vi "Read Modified.vi"(8 "error in (no error)":errorcluster, 11 "LabVIEW-Config In":refnum<class "LabVIEW-Config.lvclass">) -> (0 "error out":errorcluster, 2 "Modified?":bool, 3 "LabVIEW-Config Out":refnum<class "LabVIEW-Config.lvclass">)   [LabVIEW 2017, in "LabVIEW-Config.lvlib" / "LabVIEW-Config.lvclass"]
uses:
  LabVIEW-Config.lvclass
  LabVIEW-Config.lvclass/LabVIEW-Config.ctl
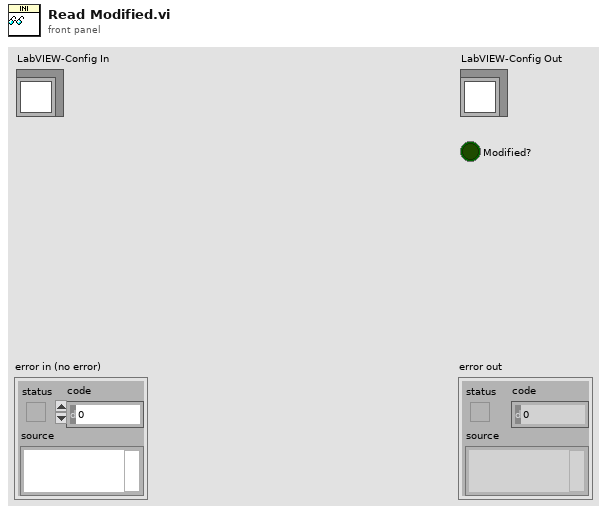
[diagram p1: front panel]
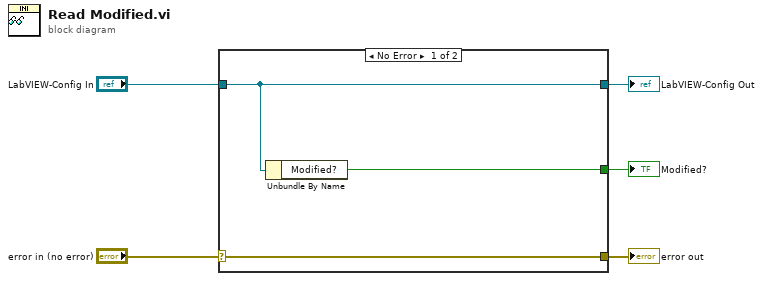
[diagram p0: block diagram]
diagram:
  n1 = case shown="No Error" "error in (no error)" {
    selector: "error in (no error)" -> [w8 w9]
    tunnel: [w8 w9] -> w4
    tunnel: [w7 w10] -> w2
    tunnel: "LabVIEW-Config In" -> [w7 w10]
    tunnel: [w6 _] -> w1
    frame No Error {
      n2 = Unbundle By Name(w7) -> ("Modified?"=w6:bool)
    }
    frame Error {
    }
  }
  "error out" <- w4
  "LabVIEW-Config Out" <- w2
  "Modified?" <- w1
